vi "motorRPS(SubVI).vi"(6 "desired rps":dbl format="%.2f", 9 "dt out (s) in":dbl, 10 "Previous Encoder Value":i32, 11 "Current Encoder Value":i32) -> (1 "rps (ride mode)":dbl, 2 "dt out (s) out":dbl, 3 "ride mode duty cycle":dbl format="%.2f")   [LabVIEW 2017]
uses:
  <vilib>/addons/control/pid/pid.llb/PID (DBL).vi
  <vilib>/addons/control/pid/NI_PID_pid.lvlib
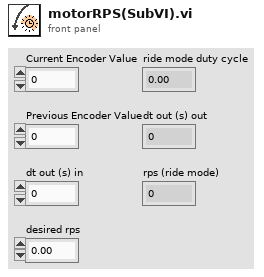
[diagram p1: front panel]
types:
  T1 = cluster{"proportional gain (Kc)":dbl, "integral time (Ti, min)":dbl, "derivative time (Td, min)":dbl}
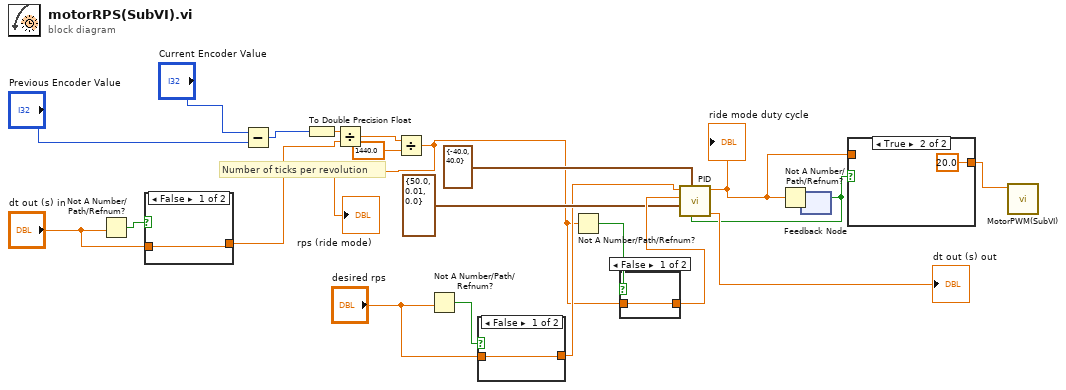
[diagram p0: block diagram]
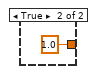
[diagram p3: hidden frame]
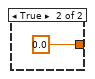
[diagram p4: hidden frame]
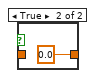
[diagram p5: hidden frame]
diagram:
  # "Number of ticks per revolution"
  n1 = Not A Number/Path/Refnum?(number/path/refnum="dt out (s) in") -> (NaN/Path/Refnum?=w7:bool)
  n2 = case shown="False" w7 {
    tunnel: "dt out (s) in" -> [w23 _]
    tunnel: [w23 1.0 ("dt out (s) in")] -> w5
    frame False {
    }
    frame True {
    }
  }
  n3 = Subtract(x="Current Encoder Value", y="Previous Encoder Value") -> (x-y=w15:i32)
  n4 = To Double Precision Float(number=w15) -> (double precision float=w16:dbl)
  n5 = Divide(x=w16, y=w5) -> (x/y=w19:dbl)
  n6 = Divide(x=w19, y=1440.0) -> (x/y=w8:dbl)
  "rps (ride mode)" <- w8
  n7 = Not A Number/Path/Refnum?(number/path/refnum="desired rps") -> (NaN/Path/Refnum?=w11:bool)
  n8 = case shown="False" w11 {
    tunnel: [w25 0.0 ("process variable")] -> w10
    tunnel: "desired rps" -> [w25 _]
    frame False {
    }
    frame True {
    }
  }
  n9 = Not A Number/Path/Refnum?(number/path/refnum=w8) -> (NaN/Path/Refnum?=w21:bool)
  n10 = case shown="False" w21 {
    tunnel: [w27 0.0 ("process variable")] -> w22
    tunnel: w8 -> [w27 _]
    frame False {
    }
    frame True {
    }
  }
  n11 = feedback #1() -> (w1:bool)  [unwired: 1 in]
  n12 = call-poly <vilib>:"PID.vi"("reinitialize? (F)"=w1, "output range"=cluster{"output high":dbl, "output low":dbl} {"output high"=-40.0, "output low"=40.0}, "PID gains"=T1 {"proportional gain (Kc)"=50.0, "integral time (Ti, min)"=0.01, "derivative time (Td, min)"=0.0}, "process variable"=w22, "setpoint"=w10) -> ("dt out (s)"=→"dt out (s) out":dbl, "output"=w4:dbl)  [unwired: 5 in]
  "ride mode duty cycle" <- w4
  n13 = Not A Number/Path/Refnum?(number/path/refnum=w4) -> (NaN/Path/Refnum?=w2:bool)
  n14 = feedback-in #1(w2) -> ()
  n15 = case shown="True" w1 {
    tunnel: w4 -> [w29 _]
    tunnel: [w29 20.0 ("output")] -> w3
    frame False {
    }
    frame True {
    }
  }
  n16 = call "MotorPWM(SubVI).vi"("Duty Cycle (-100 to + 100)"=w3) -> ()  [unwired: 11 in]
